vi "DIAdem Load Report.vi"(6 "asynchronous? (F)":bool, 7 "start path":path, 8 "error in (no error)":errorcluster, 9 "refresh report? (F)":bool, 10 "file path (dialog if empty)":path, 11 "DIAdem Reference":T1) -> (0 "error out":errorcluster, 3 "DIAdem Reference":T1)   [LabVIEW 2017]
doc: "Load the specified DIAdem layout file into the DIAdem-REPORT panel."
uses:
  <vilib>/ExportToExcel/DIAdem Reference.ctl
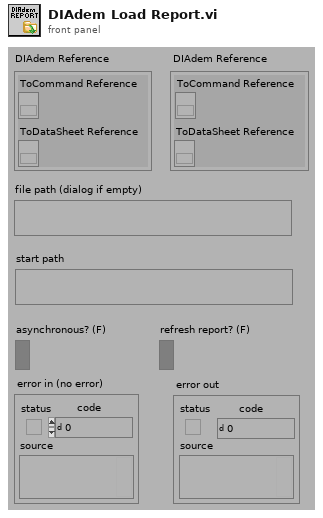
[diagram p1: front panel]
types:
  T1 = typedef "DIAdem Reference.ctl" = cluster{"ToCommand Reference":refnum<k7>, "ToDataSheet Reference":refnum<k7>}
  T2 = enum32{"existing file", "new file", "new or existing file", "existing dir", "new dir", "new or existing dir", "existing file (use LLBs)", "new file (use LLBs)", "new or existing file (use LLBs)", "new or existing file or directory (use LLBs)"}
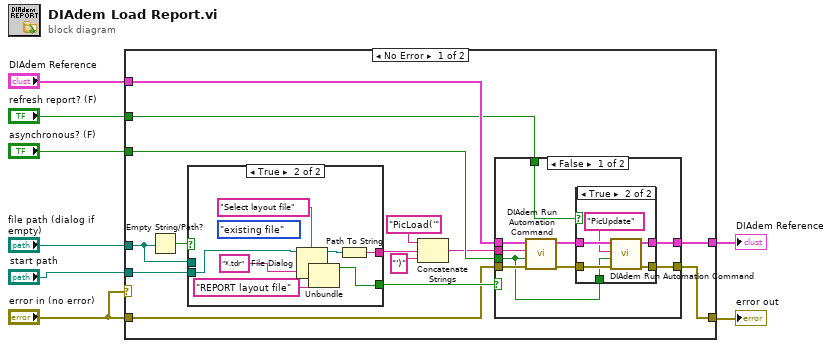
[diagram p0: block diagram]
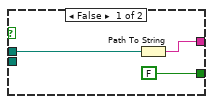
[diagram p4: hidden frame]
diagram:
  n1 = case shown="No Error" "error in (no error)" {
    tunnel: "error in (no error)" -> [w13 w54]
    tunnel: [w12 w54] -> w8
    tunnel: "DIAdem Reference" -> [w19 w53]
    tunnel: [w18 w53] -> w6
    tunnel: "file path (dialog if empty)" -> [w17 _]
    tunnel: "asynchronous? (F)" -> [w16 _]
    tunnel: "refresh report? (F)" -> [w10 _]
    tunnel: "start path" -> [w9 _]
    frame No Error {
      n2 = Empty String/Path?(string/path=w17) -> (empty?=w21:bool)
      n3 = case shown="True" w21 {
        tunnel: w17 -> [w44 _]
        tunnel: [w43 w49] -> w14
        tunnel: [FALSE ("cancelled") w48] -> w20
        tunnel: w9 -> [_ w46]
        frame False {
          n4 = Path To String(path=w44) -> (string=w43:string)
        }
        frame True {
          (unwired) T2."existing file" ("select mode (2)")
          n5 = File Dialog(4:"REPORT layout file" ("pattern label"), 6:"*.tdr" ("pattern"), 7:"Select layout file" ("prompt"), 11:w46) -> (0:w45:errorcluster, 1:w48:bool, 3:w50:path)  [unwired: 3 in, 1 out]
          n6 = Unbundle(w45) -> ()  [unwired: 3 out]
          n7 = Path To String(path=w50) -> (string=w49:string)
        }
      }
      n8 = Concatenate Strings("PicLoad('" ("Substring"), w14, "')" ("Substring")) -> (w15:string)
      n9 = case shown="False" w20 {
        tunnel: w15 -> [w31 _]
        tunnel: [w27 w40] -> w12
        tunnel: w16 -> [w24 _]
        tunnel: w19 -> [w30 w41]
        tunnel: [w28 w41] -> w18
        tunnel: w13 -> [w29 w40]
        tunnel: w10 -> [w23 _]
        frame False {
          n10 = call <vilib>:"DIAdem Run Automation Command.vi"("error in (no error)"=w29, "asynchronous? (F)"=w24, "command"=w31, "DIAdem Reference"=w30) -> ("error out"=w25:errorcluster, "DIAdem Reference"=w26:T1)  [unwired: 6 in]
          n11 = case shown="True" w23 {
            tunnel: [w33 w39] -> w28
            tunnel: [w32 w38] -> w27
            tunnel: w26 -> [w33 w37]
            tunnel: w25 -> [w32 w36]
            tunnel: w24 -> [_ w35]
            frame False {
            }
            frame True {
              n12 = call <vilib>:"DIAdem Run Automation Command.vi"("error in (no error)"=w36, "asynchronous? (F)"=w35, "command"="PicUpdate", "DIAdem Reference"=w37) -> ("error out"=w38:errorcluster, "DIAdem Reference"=w39:T1)  [unwired: 6 in]
            }
          }
        }
        frame True {
        }
      }
    }
    frame Error {
    }
  }
  "error out" <- w8
  "DIAdem Reference" <- w6
